vi "PID Reef Align.vi"(6 "Tag ID":dbl=22.0, 8 "Int per ft":dbl=0.75, 9 "setpoint":dbl=-0.575) -> (0 "PID Happy?":bool, 2 "Robot Velocities Out":cluster{"output":dbl, "y":dbl, "y":dbl}={"output"=-0.08433638301508135, "y"=1.0, "y"=0.0})   [LabVIEW 2023]
uses:
  <vilib>/Rock Robotics/WPI/DriverStation/WPI_DriverStationRobotMode2.ctl
  <vilib>/Rock Robotics/Network Tables/NT Read Numeric Array.vi
  <vilib>/Rock Robotics/Network Tables/NT Read Number.vi
  Framework/Robot Global Data.vi
  <vilib>/ptbypt/NI_PtbyPt.lvlib
panel:
  in  "Deadband Auto":dbl=0.15
  in  "Y movement":dbl=1.0
  in  "Deadband Tele":dbl=0.1
  out "Waveform Chart":cluster{"setpoint":dbl, "output":dbl}(graph)={"setpoint"=-0.5491842011911218, "output"=-0.575}
  in  "PID gains":T1={"proportional gain (Kp)"=3.3, "integral time (Ki)"=0.0, "derivative time (Kd)"=0.2} {"derivative time (Kd)" format="%.3f"; "integral time (Ki)" format="%.3f"; "proportional gain (Kp)" format="%.3f"}
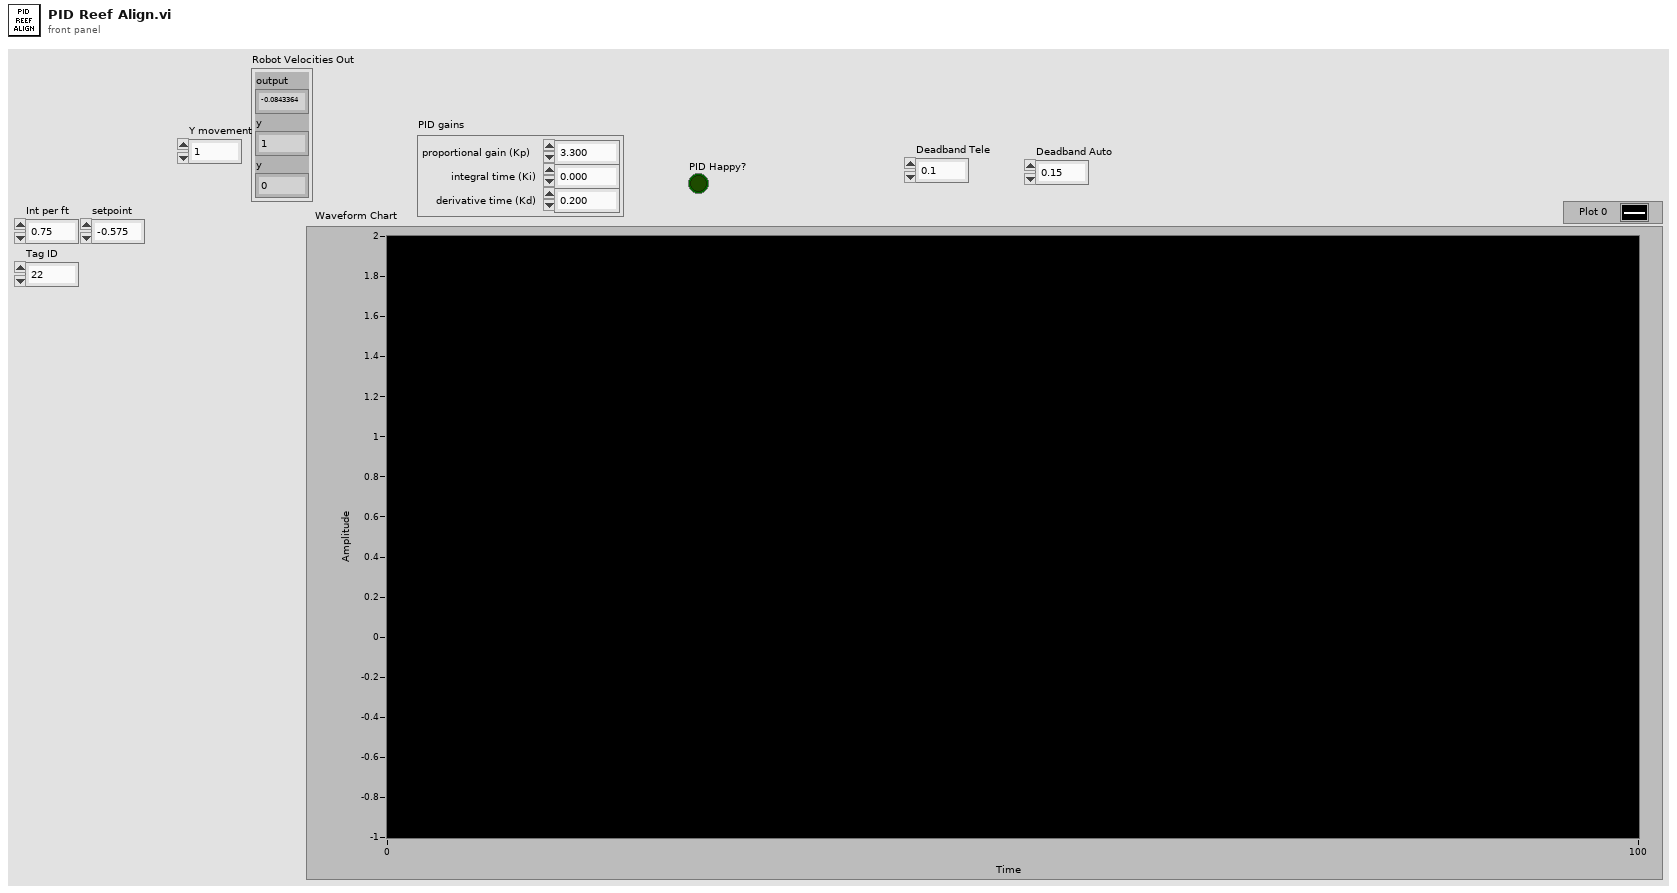
[diagram p1: front panel]
types:
  T1 = cluster{"proportional gain (Kp)":dbl, "integral time (Ki)":dbl, "derivative time (Kd)":dbl}
  T2 = typedef "WPI_DriverStationRobotMode2.ctl" = enum16{"Autonomous Disabled", "Autonomous Enabled", "Teleop Disabled", "Teleop Enabled", "Disconnected", "Finish", "Test Disabled", "Test Enabled", "Emergency Stopped"}
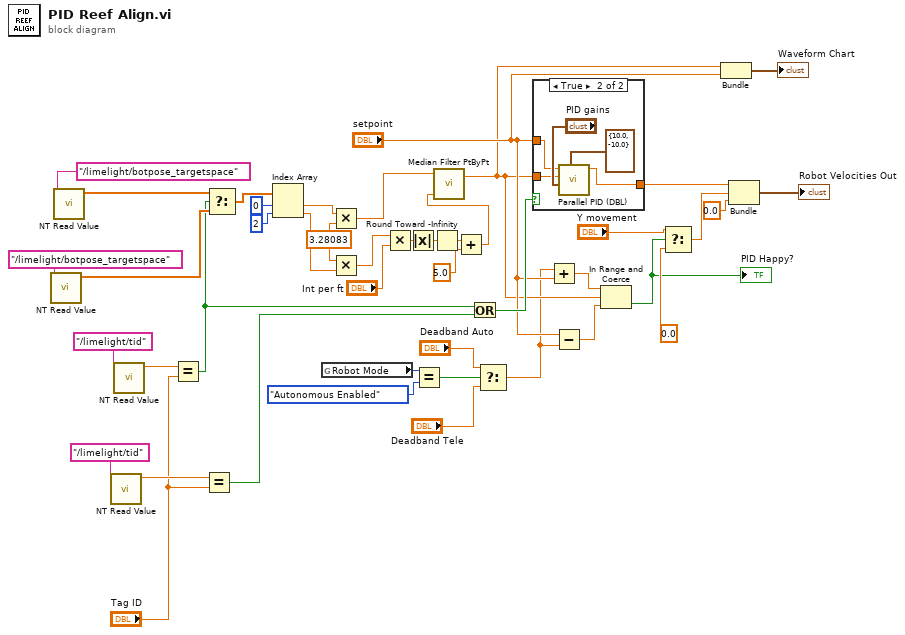
[diagram p0: block diagram]
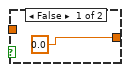
[diagram p2: hidden frame]
diagram:
  w37 = 3.28083 ("x")
  n1 = call-poly <vilib>:"NT Read Value.vi"("name"="/limelight/botpose_targetspace") -> ("value"=w27:dbl[])  [unwired: 8 in, 2 out]
  n2 = call-poly <vilib>:"NT Read Value.vi"("name"="/limelight/botpose_targetspace") -> ("value"=w28:dbl[])  [unwired: 8 in, 2 out]
  n3 = call-poly <vilib>:"NT Read Value.vi"("name"="/limelight/tid") -> ("value"=w24:dbl)  [unwired: 8 in, 2 out]
  n4 = call-poly <vilib>:"NT Read Value.vi"("name"="/limelight/tid") -> ("value"=w40:dbl)  [unwired: 8 in, 2 out]
  n5 = Equal?(x=w40, y="Tag ID") -> (x = y?=w20:bool)
  n6 = Equal?(x=w24, y="Tag ID") -> (x = y?=w21:bool)
  n7 = Select(t=w28, s=w20, f=w27) -> (s? t:f=w26:dbl[])
  n8 = Index Array(array=w26, index #1=0 ("index"), index #2=2 ("index")) -> (element #1=w42:dbl, element #2=w38:dbl)
  n9 = global read "Robot Global Data.vi" "Robot Mode"() -> (w5:T2)
  n10 = Multiply(x=w42, y=w37) -> (x*y=w18:dbl)
  n11 = Multiply(x=w37, y=w38) -> (x*y=w36:dbl)
  n12 = Multiply(x=w36, y="Int per ft") -> (x*y=w34:dbl)
  n13 = Absolute Value(x=w34) -> (abs(x)=w33:dbl)
  n14 = Equal?(x=w5, y=WPI_DriverStationRobotMode2."Autonomous Enabled") -> (x = y?=w3:bool)
  n15 = Round Toward -Infinity(1:w33) -> (0:w32:dbl)
  n16 = Add(x=w32, y=5.0) -> (x+y=w30:dbl)
  n17 = call <vilib>:"Median Filter PtByPt.vi"("rank"=w30, "x"=w18) -> ("Filtered x"=w10:dbl)  [unwired: 2 in, 1 out]
  n18 = Or(x=w20, y=w21) -> (x .or. y?=w19:bool)
  n19 = Select(t="Deadband Auto", s=w3, f="Deadband Tele") -> (s? t:f=w6:dbl)
  n20 = case shown="True" w19 {
    tunnel: w10 -> [_ w48]
    tunnel: "setpoint" -> [_ w47]
    tunnel: [0.0 ("output") w46] -> w16
    frame False {
    }
    frame True {
      n21 = call <vilib>:"Parallel PID (DBL).vi"("output range"=cluster{"high":dbl, "low":dbl} {"high"=10.0, "low"=-10.0}, "PID gains"="PID gains", "process variable"=w48, "setpoint"=w47) -> ("output"=w46:dbl)  [unwired: 4 in, 3 out]
    }
  }
  n22 = Add(x=w6, y="setpoint") -> (x+y=w13:dbl)
  n23 = Subtract(x="setpoint", y=w6) -> (x-y=w11:dbl)
  n24 = In Range and Coerce(upper limit=w13, x=w10, lower limit=w11) -> (In Range?=w7:bool)  [unwired: 1 out]
  "PID Happy?" <- w7
  n25 = Select(t="Y movement", s=w7, f=0.0) -> (s? t:f=w14:dbl)
  n26 = Bundle("Filtered x"=w10, "setpoint"="setpoint") -> (→"Waveform Chart":cluster{"Filtered x":dbl, "setpoint":dbl})  [unwired: 1 in]
  n27 = Bundle("output"=w16, "f"=w14, "y"=0.0) -> (→"Robot Velocities Out":cluster{"output":dbl, "f":dbl, "y":dbl})  [unwired: 1 in]
